vi "Write Serializer.vi"(10 "Serializer":refnum<class "Serializer.lvclass">, 11 "ConfigManager in":refnum<class "ConfigManager.lvclass">) -> (3 "ConfigManager out":refnum<class "ConfigManager.lvclass">)   [LabVIEW 2013, in "CfgManager.lvlib" / "ConfigManager.lvclass"]
uses:
  ConfigManager.lvclass
  <vilib>/LabVIEW Open Source Project/Serializer/Serializer/Serializer.lvclass
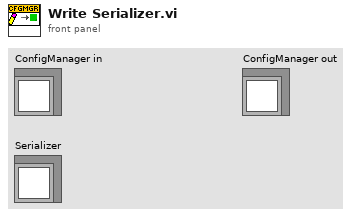
[diagram p1: front panel]
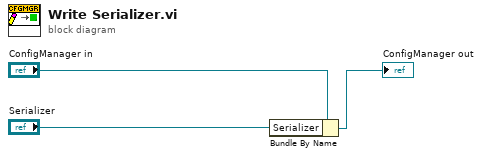
[diagram p0: block diagram]
diagram:
  n1 = Bundle By Name(cluster="ConfigManager in", "Serializer"="Serializer") -> (→"ConfigManager out":refnum<class "ConfigManager.lvclass">)
